vi "U8ArrayToSingleBigEndian(SubVI).vi"(6 "Numeric 5":u8 format="%x", 9 "Numeric 4":u8 format="%x", 10 "Numeric 3":u8 format="%x", 11 "Numeric in":u8 format="%x") -> (3 "Numeric 8":sgl)   [LabVIEW 2012]
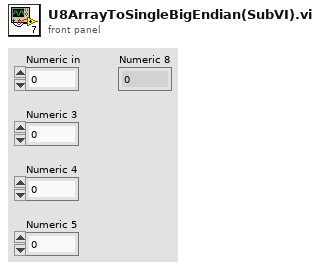
[diagram p1: front panel]
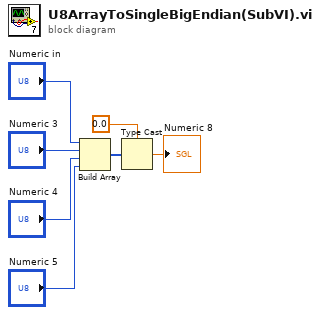
[diagram p0: block diagram]
diagram:
  n1 = Build Array("Numeric in", "Numeric 3", "Numeric 4", "Numeric 5") -> (w5:u8[])
  n2 = Type Cast(type=sgl 0.0, x=w5) -> (*(type *) &x=→"Numeric 8":sgl)
